vi "VanoceVanoce.vi"(11 "NXT/EV3":T1) -> (3 "NXT/EV3 2":T1)   [LabVIEW 2016]
uses:
  <vilib>/NXT/Subs/LVHSConnector.ctl
  <vilib>/NXT/LegoClasses/BrickReference/BrickReference.lvclass
  <vilib>/NXT/Block Support/NXT_OutputPort.ctl
  <vilib>/NXT/Dual Mode Library/Display/drawText_Center.vi
  <vilib>/NXT/Dual Mode Library/Sound/PlayC.vi
  <vilib>/NXT/Dual Mode Library/Sound/PlayA.vi
  <vilib>/NXT/Dual Mode Library/Sound/PlayG.vi
  <vilib>/NXT/Dual Mode Library/Sound/PlayE.vi
  <vilib>/NXT/Dual Mode Library/Sound/PlayD.vi
  <vilib>/NXT/Dual Mode Library/Waits/Wait_Num.vi
  <vilib>/NXT/Dual Mode Library/Sound/PlayB.vi
  <vilib>/NXT/Dual Mode Library/Sound/PlayF.vi
  <vilib>/NXT/Dual Mode Library/Sound/PlayFsharp.vi
  <vilib>/NXT/NXTIO Xnodes/NXTIONodeSubVIs/NXTMoveMotors.vi
  <vilib>/NXT/NXTIO Xnodes/NXTIONodeSubVIs/NXTStopMotors.vi
  <vilib>/NXT/NXTIO Xnodes/AddressXNode/NXTIOAddress.xnode
  <vilib>/NXT/NXTIO Xnodes/NXTIOXNode/NXTIO.xnode
panel:
  in  "Poèet opakování":i32
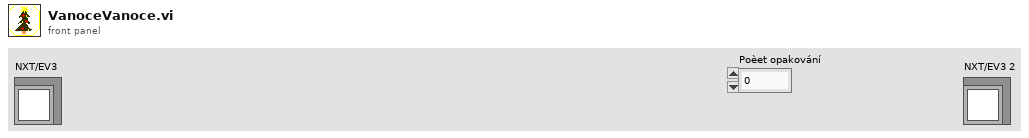
[diagram p1: front panel]
types:
  T1 = typedef "LVHSConnector.ctl" = refnum<class "BrickReference.lvclass">
  T2 = typedef "NXT_OutputPort.ctl" = u8
diagram:
  w8 = u16 5 items=["3"=3, "4"=4, "5"=5, "6"=6, "7"=7] ("Octave")
  w9 = u16 4 items=["3"=3, "4"=4, "5"=5, "6"=6, "7"=7] ("Octave")
  w10 = u16 4 items=["3"=3, "4"=4, "5"=5, "6"=6, "7"=7] ("Octave")
  w11 = u16 4 items=["3"=3, "4"=4, "5"=5, "6"=6, "7"=7] ("Octave")
  w21 = u16 4 items=["3"=3, "4"=4, "5"=5, "6"=6, "7"=7] ("Octave")
  w20 = u16 4 items=["3"=3, "4"=4, "5"=5, "6"=6, "7"=7] ("Octave")
  w48 = u16 4 items=["3"=3, "4"=4, "5"=5, "6"=6, "7"=7] ("Octave")
  w46 = u16 4 items=["3"=3, "4"=4, "5"=5, "6"=6, "7"=7] ("Octave")
  w41 = u16 4 items=["3"=3, "4"=4, "5"=5, "6"=6, "7"=7] ("Octave")
  w40 = u16 4 items=["3"=3, "4"=4, "5"=5, "6"=6, "7"=7] ("Octave")
  w35 = u16 4 items=["3"=3, "4"=4, "5"=5, "6"=6, "7"=7] ("Octave")
  w34 = u16 4 items=["3"=3, "4"=4, "5"=5, "6"=6, "7"=7] ("Octave")
  w33 = u16 4 items=["3"=3, "4"=4, "5"=5, "6"=6, "7"=7] ("Octave")
  w28 = u16 4 items=["3"=3, "4"=4, "5"=5, "6"=6, "7"=7] ("Octave")
  w25 = u16 5 items=["3"=3, "4"=4, "5"=5, "6"=6, "7"=7] ("Octave")
  w24 = u16 5 items=["3"=3, "4"=4, "5"=5, "6"=6, "7"=7] ("Octave")
  w53 = u16 4 items=["3"=3, "4"=4, "5"=5, "6"=6, "7"=7] ("Octave")
  w54 = u16 4 items=["3"=3, "4"=4, "5"=5, "6"=6, "7"=7] ("Octave")
  w55 = u16 4 items=["3"=3, "4"=4, "5"=5, "6"=6, "7"=7] ("Octave")
  w69 = u16 4 items=["3"=3, "4"=4, "5"=5, "6"=6, "7"=7] ("Octave")
  w70 = u16 4 items=["3"=3, "4"=4, "5"=5, "6"=6, "7"=7] ("Octave")
  w71 = u16 4 items=["3"=3, "4"=4, "5"=5, "6"=6, "7"=7] ("Octave")
  w72 = u16 4 items=["3"=3, "4"=4, "5"=5, "6"=6, "7"=7] ("Octave")
  w73 = u16 4 items=["3"=3, "4"=4, "5"=5, "6"=6, "7"=7] ("Octave")
  w74 = u16 4 items=["3"=3, "4"=4, "5"=5, "6"=6, "7"=7] ("Octave")
  w86 = u16 4 items=["3"=3, "4"=4, "5"=5, "6"=6, "7"=7] ("Octave")
  w88 = u16 4 items=["3"=3, "4"=4, "5"=5, "6"=6, "7"=7] ("Octave")
  w93 = u16 4 items=["3"=3, "4"=4, "5"=5, "6"=6, "7"=7] ("Octave")
  w94 = u16 4 items=["3"=3, "4"=4, "5"=5, "6"=6, "7"=7] ("Octave")
  w99 = u16 4 items=["3"=3, "4"=4, "5"=5, "6"=6, "7"=7] ("Octave")
  w100 = u16 4 items=["3"=3, "4"=4, "5"=5, "6"=6, "7"=7] ("Octave")
  w101 = u16 4 items=["3"=3, "4"=4, "5"=5, "6"=6, "7"=7] ("Octave")
  w107 = u16 4 items=["3"=3, "4"=4, "5"=5, "6"=6, "7"=7] ("Octave")
  w110 = u16 5 items=["3"=3, "4"=4, "5"=5, "6"=6, "7"=7] ("Octave")
  w111 = u16 5 items=["3"=3, "4"=4, "5"=5, "6"=6, "7"=7] ("Octave")
  w116 = u16 4 items=["3"=3, "4"=4, "5"=5, "6"=6, "7"=7] ("Octave")
  w119 = u16 4 items=["3"=3, "4"=4, "5"=5, "6"=6, "7"=7] ("Octave")
  w120 = u16 4 items=["3"=3, "4"=4, "5"=5, "6"=6, "7"=7] ("Octave")
  w146 = u16 4 items=["3"=3, "4"=4, "5"=5, "6"=6, "7"=7] ("Octave")
  w150 = u16 4 items=["3"=3, "4"=4, "5"=5, "6"=6, "7"=7] ("Octave")
  w147 = u16 4 items=["3"=3, "4"=4, "5"=5, "6"=6, "7"=7] ("Octave")
  w139 = u16 4 items=["3"=3, "4"=4, "5"=5, "6"=6, "7"=7] ("Octave")
  w136 = u16 4 items=["3"=3, "4"=4, "5"=5, "6"=6, "7"=7] ("Octave")
  w131 = u16 4 items=["3"=3, "4"=4, "5"=5, "6"=6, "7"=7] ("Octave")
  w134 = u16 4 items=["3"=3, "4"=4, "5"=5, "6"=6, "7"=7] ("Octave")
  w126 = u16 4 items=["3"=3, "4"=4, "5"=5, "6"=6, "7"=7] ("Octave")
  w123 = u16 4 items=["3"=3, "4"=4, "5"=5, "6"=6, "7"=7] ("Octave")
  w122 = u16 4 items=["3"=3, "4"=4, "5"=5, "6"=6, "7"=7] ("Octave")
  w168 = u16 4 items=["3"=3, "4"=4, "5"=5, "6"=6, "7"=7] ("Octave")
  w165 = u16 4 items=["3"=3, "4"=4, "5"=5, "6"=6, "7"=7] ("Octave")
  w161 = u16 4 items=["3"=3, "4"=4, "5"=5, "6"=6, "7"=7] ("Octave")
  w164 = u16 4 items=["3"=3, "4"=4, "5"=5, "6"=6, "7"=7] ("Octave")
  w176 = u16 4 items=["3"=3, "4"=4, "5"=5, "6"=6, "7"=7] ("Octave")
  w179 = u16 4 items=["3"=3, "4"=4, "5"=5, "6"=6, "7"=7] ("Octave")
  w184 = u16 4 items=["3"=3, "4"=4, "5"=5, "6"=6, "7"=7] ("Octave")
  w181 = u16 4 items=["3"=3, "4"=4, "5"=5, "6"=6, "7"=7] ("Octave")
  w189 = u16 4 items=["3"=3, "4"=4, "5"=5, "6"=6, "7"=7] ("Octave")
  w192 = u16 4 items=["3"=3, "4"=4, "5"=5, "6"=6, "7"=7] ("Octave")
  w193 = u16 4 items=["3"=3, "4"=4, "5"=5, "6"=6, "7"=7] ("Octave")
  w196 = u16 4 items=["3"=3, "4"=4, "5"=5, "6"=6, "7"=7] ("Octave")
  w204 = u16 5 items=["3"=3, "4"=4, "5"=5, "6"=6, "7"=7] ("Octave")
  w205 = u16 4 items=["3"=3, "4"=4, "5"=5, "6"=6, "7"=7] ("Octave")
  w206 = u16 4 items=["3"=3, "4"=4, "5"=5, "6"=6, "7"=7] ("Octave")
  w207 = u16 4 items=["3"=3, "4"=4, "5"=5, "6"=6, "7"=7] ("Octave")
  w217 = u16 4 items=["3"=3, "4"=4, "5"=5, "6"=6, "7"=7] ("Octave")
  w216 = u16 4 items=["3"=3, "4"=4, "5"=5, "6"=6, "7"=7] ("Octave")
  w244 = u16 4 items=["3"=3, "4"=4, "5"=5, "6"=6, "7"=7] ("Octave")
  w242 = u16 4 items=["3"=3, "4"=4, "5"=5, "6"=6, "7"=7] ("Octave")
  w237 = u16 4 items=["3"=3, "4"=4, "5"=5, "6"=6, "7"=7] ("Octave")
  w236 = u16 4 items=["3"=3, "4"=4, "5"=5, "6"=6, "7"=7] ("Octave")
  w231 = u16 4 items=["3"=3, "4"=4, "5"=5, "6"=6, "7"=7] ("Octave")
  w230 = u16 4 items=["3"=3, "4"=4, "5"=5, "6"=6, "7"=7] ("Octave")
  w229 = u16 4 items=["3"=3, "4"=4, "5"=5, "6"=6, "7"=7] ("Octave")
  w224 = u16 4 items=["3"=3, "4"=4, "5"=5, "6"=6, "7"=7] ("Octave")
  w221 = u16 5 items=["3"=3, "4"=4, "5"=5, "6"=6, "7"=7] ("Octave")
  w220 = u16 5 items=["3"=3, "4"=4, "5"=5, "6"=6, "7"=7] ("Octave")
  w249 = u16 4 items=["3"=3, "4"=4, "5"=5, "6"=6, "7"=7] ("Octave")
  w250 = u16 4 items=["3"=3, "4"=4, "5"=5, "6"=6, "7"=7] ("Octave")
  w251 = u16 4 items=["3"=3, "4"=4, "5"=5, "6"=6, "7"=7] ("Octave")
  w265 = u16 4 items=["3"=3, "4"=4, "5"=5, "6"=6, "7"=7] ("Octave")
  w266 = u16 4 items=["3"=3, "4"=4, "5"=5, "6"=6, "7"=7] ("Octave")
  w267 = u16 4 items=["3"=3, "4"=4, "5"=5, "6"=6, "7"=7] ("Octave")
  w268 = u16 4 items=["3"=3, "4"=4, "5"=5, "6"=6, "7"=7] ("Octave")
  w269 = u16 4 items=["3"=3, "4"=4, "5"=5, "6"=6, "7"=7] ("Octave")
  w270 = u16 4 items=["3"=3, "4"=4, "5"=5, "6"=6, "7"=7] ("Octave")
  w280 = i16 5 items=["1", "2", "3", "4", "5", "6", "7", "8", "9", "10", "11", "12"] ("Line")
  w284 = u16 4 items=["3"=3, "4"=4, "5"=5, "6"=6, "7"=7] ("Octave")
  w286 = u16 4 items=["3"=3, "4"=4, "5"=5, "6"=6, "7"=7] ("Octave")
  w291 = u16 4 items=["3"=3, "4"=4, "5"=5, "6"=6, "7"=7] ("Octave")
  w292 = u16 4 items=["3"=3, "4"=4, "5"=5, "6"=6, "7"=7] ("Octave")
  w297 = u16 4 items=["3"=3, "4"=4, "5"=5, "6"=6, "7"=7] ("Octave")
  w298 = u16 4 items=["3"=3, "4"=4, "5"=5, "6"=6, "7"=7] ("Octave")
  w299 = u16 4 items=["3"=3, "4"=4, "5"=5, "6"=6, "7"=7] ("Octave")
  w305 = u16 4 items=["3"=3, "4"=4, "5"=5, "6"=6, "7"=7] ("Octave")
  w308 = u16 5 items=["3"=3, "4"=4, "5"=5, "6"=6, "7"=7] ("Octave")
  w309 = u16 5 items=["3"=3, "4"=4, "5"=5, "6"=6, "7"=7] ("Octave")
  n1 = for {
    N: "Poèet opakování" -> [_]
    n2 = xnode "Motors"() -> ("Motor"=w313:cluster{"Port":T2, "Port":T2})
    n3 = xnode "Move Motors"("Power/Speed 2"=i8 -75, "Power/Speed 1"=i8 75, "Motors"=w313) -> ("NXT/EV3"=w328:T1)  [unwired: 1 in]
    n4 = call-poly <vilib>:"PolyWait.vi"("Time (1 sec)"=sgl 0.5, "NXT/EV3"=w328) -> ("NXT/EV3"=w327:T1)  [unwired: 2 in]
    n5 = xnode "Stop Motors"("Motors"=w313, "NXT/EV3"=w327) -> ("NXT/EV3"=w319:T1)
    n6 = xnode "Move Motors"("Power/Speed 2"=i8 75, "Power/Speed 1"=i8 -75, "Motors"=w313, "NXT/EV3"=w319) -> ("NXT/EV3"=w320:T1)
    n7 = call-poly <vilib>:"PolyWait.vi"("Time (1 sec)"=sgl 0.5, "NXT/EV3"=w320) -> ("NXT/EV3"=w321:T1)  [unwired: 2 in]
    n8 = xnode "Stop Motors"("Motors"=w313, "NXT/EV3"=w321) -> ("NXT/EV3"=w312:T1)
    n9 = xnode "Move Motors"("Power/Speed 2"=i8 20, "Power/Speed 1"=i8 20, "Motors"=w313, "NXT/EV3"=w312) -> ("NXT/EV3"=w317:T1)
    n10 = call-poly <vilib>:"PolyWait.vi"("Time (1 sec)"=sgl 0.5, "NXT/EV3"=w317) -> ("NXT/EV3"=w316:T1)  [unwired: 2 in]
    n11 = xnode "Stop Motors"("Motors"=w313, "NXT/EV3"=w316) -> ()  [unwired: 1 out]
  }
  n12 = call-poly <vilib>:"PolyDisplay.vi"("Text"="EV3 JUK3BOX:\nVanoce, Vanoce\n", "NXT/EV3"="NXT/EV3", "Line"=w280) -> ("NXT/EV3"=w197:T1)  [unwired: 1 in]
  n13 = call-poly <vilib>:"PolySound.vi"("Duration (500 ms)"=u16 1000, "NXT/EV3"=w197, "Octave"=w309) -> ("NXT/EV3"=w304:T1)  [unwired: 1 in]
  n14 = call-poly <vilib>:"PolySound.vi"("Duration (500 ms)"=u16 500, "NXT/EV3"=w304, "Octave"=w308) -> ("NXT/EV3"=w303:T1)  [unwired: 1 in]
  n15 = call-poly <vilib>:"PolySound.vi"("Duration (500 ms)"=u16 500, "NXT/EV3"=w303, "Octave"=w305) -> ("NXT/EV3"=w302:T1)  [unwired: 1 in]
  n16 = call-poly <vilib>:"PolySound.vi"("Duration (500 ms)"=u16 1000, "NXT/EV3"=w302, "Octave"=w299) -> ("NXT/EV3"=w301:T1)  [unwired: 1 in]
  n17 = call-poly <vilib>:"PolySound.vi"("Duration (500 ms)"=u16 500, "NXT/EV3"=w301, "Octave"=w298) -> ("NXT/EV3"=w300:T1)  [unwired: 1 in]
  n18 = call-poly <vilib>:"PolySound.vi"("Duration (500 ms)"=u16 500, "NXT/EV3"=w300, "Octave"=w297) -> ("NXT/EV3"=w289:T1)  [unwired: 1 in]
  n19 = call-poly <vilib>:"PolySound.vi"("Duration (500 ms)"=u16 500, "NXT/EV3"=w289, "Octave"=w292) -> ("NXT/EV3"=w288:T1)  [unwired: 1 in]
  n20 = call-poly <vilib>:"PolySound.vi"("Duration (500 ms)"=u16 1000, "NXT/EV3"=w288, "Octave"=w291) -> ("NXT/EV3"=w285:T1)  [unwired: 1 in]
  n21 = call-poly <vilib>:"PolySound.vi"("Duration (500 ms)"=u16 500, "NXT/EV3"=w285, "Octave"=w286) -> ("NXT/EV3"=w283:T1)  [unwired: 1 in]
  n22 = call-poly <vilib>:"PolySound.vi"("Duration (500 ms)"=u16 1000, "NXT/EV3"=w283, "Octave"=w284) -> ("NXT/EV3"=w262:T1)  [unwired: 1 in]
  n23 = call-poly <vilib>:"PolyWait.vi"("Time (1 sec)"=sgl 0.7, "NXT/EV3"=w262) -> ("NXT/EV3"=w261:T1)  [unwired: 2 in]
  n24 = call-poly <vilib>:"PolySound.vi"("Duration (500 ms)"=u16 500, "NXT/EV3"=w261, "Octave"=w270) -> ("NXT/EV3"=w279:T1)  [unwired: 1 in]
  n25 = call-poly <vilib>:"PolySound.vi"("Duration (500 ms)"=u16 1000, "NXT/EV3"=w279, "Octave"=w269) -> ("NXT/EV3"=w278:T1)  [unwired: 1 in]
  n26 = call-poly <vilib>:"PolySound.vi"("Duration (500 ms)"=u16 500, "NXT/EV3"=w278, "Octave"=w268) -> ("NXT/EV3"=w277:T1)  [unwired: 1 in]
  n27 = call-poly <vilib>:"PolySound.vi"("Duration (500 ms)"=u16 1000, "NXT/EV3"=w277, "Octave"=w267) -> ("NXT/EV3"=w276:T1)  [unwired: 1 in]
  n28 = call-poly <vilib>:"PolySound.vi"("Duration (500 ms)"=u16 1000, "NXT/EV3"=w276, "Octave"=w266) -> ("NXT/EV3"=w263:T1)  [unwired: 1 in]
  n29 = call-poly <vilib>:"PolySound.vi"("Duration (500 ms)"=u16 1900, "NXT/EV3"=w263, "Octave"=w265) -> ("NXT/EV3"=w259:T1)  [unwired: 1 in]
  n30 = call-poly <vilib>:"PolyWait.vi"("Time (1 sec)"=sgl 0.3, "NXT/EV3"=w259) -> ("NXT/EV3"=w257:T1)  [unwired: 2 in]
  n31 = call-poly <vilib>:"PolySound.vi"("Duration (500 ms)"=u16 500, "NXT/EV3"=w257, "Octave"=w251) -> ("NXT/EV3"=w256:T1)  [unwired: 1 in]
  n32 = call-poly <vilib>:"PolySound.vi"("Duration (500 ms)"=u16 500, "NXT/EV3"=w256, "Octave"=w250) -> ("NXT/EV3"=w255:T1)  [unwired: 1 in]
  n33 = call-poly <vilib>:"PolySound.vi"("Duration (500 ms)"=u16 500, "NXT/EV3"=w255, "Octave"=w249) -> ("NXT/EV3"=w218:T1)  [unwired: 1 in]
  n34 = call-poly <vilib>:"PolySound.vi"("Duration (500 ms)"=u16 1000, "NXT/EV3"=w218, "Octave"=w220) -> ("NXT/EV3"=w225:T1)  [unwired: 1 in]
  n35 = call-poly <vilib>:"PolySound.vi"("Duration (500 ms)"=u16 500, "NXT/EV3"=w225, "Octave"=w221) -> ("NXT/EV3"=w198:T1)  [unwired: 1 in]
  "NXT/EV3 2" <- w198
  n36 = call-poly <vilib>:"PolySound.vi"("Duration (500 ms)"=u16 500, "NXT/EV3"=w198, "Octave"=w224) -> ("NXT/EV3"=w226:T1)  [unwired: 1 in]
  n37 = call-poly <vilib>:"PolySound.vi"("Duration (500 ms)"=u16 1000, "NXT/EV3"=w226, "Octave"=w229) -> ("NXT/EV3"=w227:T1)  [unwired: 1 in]
  n38 = call-poly <vilib>:"PolySound.vi"("Duration (500 ms)"=u16 500, "NXT/EV3"=w227, "Octave"=w230) -> ("NXT/EV3"=w228:T1)  [unwired: 1 in]
  n39 = call-poly <vilib>:"PolySound.vi"("Duration (500 ms)"=u16 500, "NXT/EV3"=w228, "Octave"=w231) -> ("NXT/EV3"=w239:T1)  [unwired: 1 in]
  n40 = call-poly <vilib>:"PolySound.vi"("Duration (500 ms)"=u16 500, "NXT/EV3"=w239, "Octave"=w236) -> ("NXT/EV3"=w240:T1)  [unwired: 1 in]
  n41 = call-poly <vilib>:"PolySound.vi"("Duration (500 ms)"=u16 1000, "NXT/EV3"=w240, "Octave"=w237) -> ("NXT/EV3"=w243:T1)  [unwired: 1 in]
  n42 = call-poly <vilib>:"PolySound.vi"("Duration (500 ms)"=u16 500, "NXT/EV3"=w243, "Octave"=w242) -> ("NXT/EV3"=w245:T1)  [unwired: 1 in]
  n43 = call-poly <vilib>:"PolySound.vi"("Duration (500 ms)"=u16 1000, "NXT/EV3"=w245, "Octave"=w244) -> ("NXT/EV3"=w247:T1)  [unwired: 1 in]
  n44 = call-poly <vilib>:"PolyWait.vi"("Time (1 sec)"=sgl 0.7, "NXT/EV3"=w247) -> ("NXT/EV3"=w212:T1)  [unwired: 2 in]
  n45 = call-poly <vilib>:"PolySound.vi"("Duration (500 ms)"=u16 500, "NXT/EV3"=w212, "Octave"=w216) -> ("NXT/EV3"=w213:T1)  [unwired: 1 in]
  n46 = call-poly <vilib>:"PolySound.vi"("Duration (500 ms)"=u16 1000, "NXT/EV3"=w213, "Octave"=w217) -> ("NXT/EV3"=w211:T1)  [unwired: 1 in]
  n47 = call-poly <vilib>:"PolySound.vi"("Duration (500 ms)"=u16 500, "NXT/EV3"=w211, "Octave"=w207) -> ("NXT/EV3"=w210:T1)  [unwired: 1 in]
  n48 = call-poly <vilib>:"PolySound.vi"("Duration (500 ms)"=u16 1000, "NXT/EV3"=w210, "Octave"=w206) -> ("NXT/EV3"=w209:T1)  [unwired: 1 in]
  n49 = call-poly <vilib>:"PolySound.vi"("Duration (500 ms)"=u16 1000, "NXT/EV3"=w209, "Octave"=w205) -> ("NXT/EV3"=w208:T1)  [unwired: 1 in]
  n50 = call-poly <vilib>:"PolySound.vi"("Duration (500 ms)"=u16 2000, "NXT/EV3"=w208, "Octave"=w204) -> ("NXT/EV3"=w173:T1)  [unwired: 1 in]
  n51 = call-poly <vilib>:"PolyWait.vi"("Time (1 sec)"=sgl 0.7, "NXT/EV3"=w173) -> ("NXT/EV3"=w172:T1)  [unwired: 2 in]
  n52 = call-poly <vilib>:"PolySound.vi"("Duration (500 ms)"=u16 500, "NXT/EV3"=w172, "Octave"=w196) -> ("NXT/EV3"=w188:T1)  [unwired: 1 in]
  n53 = call-poly <vilib>:"PolySound.vi"("Duration (500 ms)"=u16 500, "NXT/EV3"=w188, "Octave"=w193) -> ("NXT/EV3"=w187:T1)  [unwired: 1 in]
  n54 = call-poly <vilib>:"PolySound.vi"("Duration (500 ms)"=u16 500, "NXT/EV3"=w187, "Octave"=w192) -> ("NXT/EV3"=w186:T1)  [unwired: 1 in]
  n55 = call-poly <vilib>:"PolySound.vi"("Duration (500 ms)"=u16 500, "NXT/EV3"=w186, "Octave"=w189) -> ("NXT/EV3"=w180:T1)  [unwired: 1 in]
  n56 = call-poly <vilib>:"PolySound.vi"("Duration (500 ms)"=u16 500, "NXT/EV3"=w180, "Octave"=w181) -> ("NXT/EV3"=w185:T1)  [unwired: 1 in]
  n57 = call-poly <vilib>:"PolySound.vi"("Duration (500 ms)"=u16 500, "NXT/EV3"=w185, "Octave"=w184) -> ("NXT/EV3"=w174:T1)  [unwired: 1 in]
  n58 = call-poly <vilib>:"PolySound.vi"("Duration (500 ms)"=u16 500, "NXT/EV3"=w174, "Octave"=w179) -> ("NXT/EV3"=w175:T1)  [unwired: 1 in]
  n59 = call-poly <vilib>:"PolySound.vi"("Duration (500 ms)"=u16 500, "NXT/EV3"=w175, "Octave"=w176) -> ("NXT/EV3"=w159:T1)  [unwired: 1 in]
  n60 = call-poly <vilib>:"PolySound.vi"("Duration (500 ms)"=u16 500, "NXT/EV3"=w159, "Octave"=w164) -> ("NXT/EV3"=w160:T1)  [unwired: 1 in]
  n61 = call-poly <vilib>:"PolySound.vi"("Duration (500 ms)"=u16 500, "NXT/EV3"=w160, "Octave"=w161) -> ("NXT/EV3"=w170:T1)  [unwired: 1 in]
  n62 = call-poly <vilib>:"PolySound.vi"("Duration (500 ms)"=u16 500, "NXT/EV3"=w170, "Octave"=w165) -> ("NXT/EV3"=w169:T1)  [unwired: 1 in]
  n63 = call-poly <vilib>:"PolySound.vi"("Duration (500 ms)"=u16 500, "NXT/EV3"=w169, "Octave"=w168) -> ("NXT/EV3"=w158:T1)  [unwired: 1 in]
  n64 = call-poly <vilib>:"PolySound.vi"("Duration (500 ms)"=u16 500, "NXT/EV3"=w158) -> ("NXT/EV3"=w157:T1)  [unwired: 2 in]
  n65 = call-poly <vilib>:"PolySound.vi"("Duration (500 ms)"=u16 500, "NXT/EV3"=w157) -> ("NXT/EV3"=w156:T1)  [unwired: 2 in]
  n66 = call-poly <vilib>:"PolySound.vi"("Duration (500 ms)"=u16 750, "NXT/EV3"=w156) -> ("NXT/EV3"=w118:T1)  [unwired: 2 in]
  n67 = call-poly <vilib>:"PolySound.vi"("NXT/EV3"=w118, "Octave"=w119) -> ("NXT/EV3"=w127:T1)  [unwired: 2 in]
  n68 = call-poly <vilib>:"PolySound.vi"("Duration (500 ms)"=u16 500, "NXT/EV3"=w127, "Octave"=w122) -> ("NXT/EV3"=w128:T1)  [unwired: 1 in]
  n69 = call-poly <vilib>:"PolySound.vi"("Duration (500 ms)"=u16 500, "NXT/EV3"=w128, "Octave"=w123) -> ("NXT/EV3"=w129:T1)  [unwired: 1 in]
  n70 = call-poly <vilib>:"PolySound.vi"("Duration (500 ms)"=u16 500, "NXT/EV3"=w129, "Octave"=w126) -> ("NXT/EV3"=w135:T1)  [unwired: 1 in]
  n71 = call-poly <vilib>:"PolySound.vi"("Duration (500 ms)"=u16 500, "NXT/EV3"=w135, "Octave"=w134) -> ("NXT/EV3"=w130:T1)  [unwired: 1 in]
  n72 = call-poly <vilib>:"PolySound.vi"("Duration (500 ms)"=u16 500, "NXT/EV3"=w130, "Octave"=w131) -> ("NXT/EV3"=w141:T1)  [unwired: 1 in]
  n73 = call-poly <vilib>:"PolySound.vi"("Duration (500 ms)"=u16 500, "NXT/EV3"=w141, "Octave"=w136) -> ("NXT/EV3"=w140:T1)  [unwired: 1 in]
  n74 = call-poly <vilib>:"PolySound.vi"("Duration (500 ms)"=u16 500, "NXT/EV3"=w140, "Octave"=w139) -> ("NXT/EV3"=w152:T1)  [unwired: 1 in]
  n75 = call-poly <vilib>:"PolySound.vi"("Duration (500 ms)"=u16 500, "NXT/EV3"=w152, "Octave"=w147) -> ("NXT/EV3"=w151:T1)  [unwired: 1 in]
  n76 = call-poly <vilib>:"PolySound.vi"("Duration (500 ms)"=u16 500, "NXT/EV3"=w151, "Octave"=w150) -> ("NXT/EV3"=w142:T1)  [unwired: 1 in]
  n77 = call-poly <vilib>:"PolySound.vi"("Duration (500 ms)"=u16 500, "NXT/EV3"=w142, "Octave"=w146) -> ("NXT/EV3"=w143:T1)  [unwired: 1 in]
  n78 = call-poly <vilib>:"PolySound.vi"("Duration (500 ms)"=u16 500, "NXT/EV3"=w143, "Octave"=w120) -> ("NXT/EV3"=w115:T1)  [unwired: 1 in]
  n79 = call-poly <vilib>:"PolySound.vi"("Duration (500 ms)"=u16 750, "NXT/EV3"=w115, "Octave"=w116) -> ("NXT/EV3"=w114:T1)  [unwired: 1 in]
  n80 = call-poly <vilib>:"PolyWait.vi"("Time (1 sec)"=sgl 0.75, "NXT/EV3"=w114) -> ("NXT/EV3"=w2:T1)  [unwired: 2 in]
  n81 = call-poly <vilib>:"PolySound.vi"("Duration (500 ms)"=u16 1000, "NXT/EV3"=w2, "Octave"=w111) -> ("NXT/EV3"=w106:T1)  [unwired: 1 in]
  n82 = call-poly <vilib>:"PolySound.vi"("Duration (500 ms)"=u16 500, "NXT/EV3"=w106, "Octave"=w110) -> ("NXT/EV3"=w105:T1)  [unwired: 1 in]
  n83 = call-poly <vilib>:"PolySound.vi"("Duration (500 ms)"=u16 500, "NXT/EV3"=w105, "Octave"=w107) -> ("NXT/EV3"=w104:T1)  [unwired: 1 in]
  n84 = call-poly <vilib>:"PolySound.vi"("Duration (500 ms)"=u16 1000, "NXT/EV3"=w104, "Octave"=w101) -> ("NXT/EV3"=w103:T1)  [unwired: 1 in]
  n85 = call-poly <vilib>:"PolySound.vi"("Duration (500 ms)"=u16 500, "NXT/EV3"=w103, "Octave"=w100) -> ("NXT/EV3"=w102:T1)  [unwired: 1 in]
  n86 = call-poly <vilib>:"PolySound.vi"("Duration (500 ms)"=u16 500, "NXT/EV3"=w102, "Octave"=w99) -> ("NXT/EV3"=w91:T1)  [unwired: 1 in]
  n87 = call-poly <vilib>:"PolySound.vi"("Duration (500 ms)"=u16 500, "NXT/EV3"=w91, "Octave"=w94) -> ("NXT/EV3"=w90:T1)  [unwired: 1 in]
  n88 = call-poly <vilib>:"PolySound.vi"("Duration (500 ms)"=u16 1000, "NXT/EV3"=w90, "Octave"=w93) -> ("NXT/EV3"=w87:T1)  [unwired: 1 in]
  n89 = call-poly <vilib>:"PolySound.vi"("Duration (500 ms)"=u16 500, "NXT/EV3"=w87, "Octave"=w88) -> ("NXT/EV3"=w85:T1)  [unwired: 1 in]
  n90 = call-poly <vilib>:"PolySound.vi"("Duration (500 ms)"=u16 1000, "NXT/EV3"=w85, "Octave"=w86) -> ("NXT/EV3"=w66:T1)  [unwired: 1 in]
  n91 = call-poly <vilib>:"PolyWait.vi"("Time (1 sec)"=sgl 0.7, "NXT/EV3"=w66) -> ("NXT/EV3"=w65:T1)  [unwired: 2 in]
  n92 = call-poly <vilib>:"PolySound.vi"("Duration (500 ms)"=u16 500, "NXT/EV3"=w65, "Octave"=w74) -> ("NXT/EV3"=w83:T1)  [unwired: 1 in]
  n93 = call-poly <vilib>:"PolySound.vi"("Duration (500 ms)"=u16 1000, "NXT/EV3"=w83, "Octave"=w73) -> ("NXT/EV3"=w82:T1)  [unwired: 1 in]
  n94 = call-poly <vilib>:"PolySound.vi"("Duration (500 ms)"=u16 500, "NXT/EV3"=w82, "Octave"=w72) -> ("NXT/EV3"=w81:T1)  [unwired: 1 in]
  n95 = call-poly <vilib>:"PolySound.vi"("Duration (500 ms)"=u16 1000, "NXT/EV3"=w81, "Octave"=w71) -> ("NXT/EV3"=w80:T1)  [unwired: 1 in]
  n96 = call-poly <vilib>:"PolySound.vi"("Duration (500 ms)"=u16 1000, "NXT/EV3"=w80, "Octave"=w70) -> ("NXT/EV3"=w67:T1)  [unwired: 1 in]
  n97 = call-poly <vilib>:"PolySound.vi"("Duration (500 ms)"=u16 1900, "NXT/EV3"=w67, "Octave"=w69) -> ("NXT/EV3"=w63:T1)  [unwired: 1 in]
  n98 = call-poly <vilib>:"PolyWait.vi"("Time (1 sec)"=sgl 0.3, "NXT/EV3"=w63) -> ("NXT/EV3"=w61:T1)  [unwired: 2 in]
  n99 = call-poly <vilib>:"PolySound.vi"("Duration (500 ms)"=u16 500, "NXT/EV3"=w61, "Octave"=w55) -> ("NXT/EV3"=w60:T1)  [unwired: 1 in]
  n100 = call-poly <vilib>:"PolySound.vi"("Duration (500 ms)"=u16 500, "NXT/EV3"=w60, "Octave"=w54) -> ("NXT/EV3"=w59:T1)  [unwired: 1 in]
  n101 = call-poly <vilib>:"PolySound.vi"("Duration (500 ms)"=u16 500, "NXT/EV3"=w59, "Octave"=w53) -> ("NXT/EV3"=w22:T1)  [unwired: 1 in]
  n102 = call-poly <vilib>:"PolySound.vi"("Duration (500 ms)"=u16 1000, "NXT/EV3"=w22, "Octave"=w24) -> ("NXT/EV3"=w29:T1)  [unwired: 1 in]
  n103 = call-poly <vilib>:"PolySound.vi"("Duration (500 ms)"=u16 500, "NXT/EV3"=w29, "Octave"=w25) -> ("NXT/EV3"=w3:T1)  [unwired: 1 in]
  n104 = call-poly <vilib>:"PolySound.vi"("Duration (500 ms)"=u16 500, "NXT/EV3"=w3, "Octave"=w28) -> ("NXT/EV3"=w30:T1)  [unwired: 1 in]
  n105 = call-poly <vilib>:"PolySound.vi"("Duration (500 ms)"=u16 1000, "NXT/EV3"=w30, "Octave"=w33) -> ("NXT/EV3"=w31:T1)  [unwired: 1 in]
  n106 = call-poly <vilib>:"PolySound.vi"("Duration (500 ms)"=u16 500, "NXT/EV3"=w31, "Octave"=w34) -> ("NXT/EV3"=w32:T1)  [unwired: 1 in]
  n107 = call-poly <vilib>:"PolySound.vi"("Duration (500 ms)"=u16 500, "NXT/EV3"=w32, "Octave"=w35) -> ("NXT/EV3"=w43:T1)  [unwired: 1 in]
  n108 = call-poly <vilib>:"PolySound.vi"("Duration (500 ms)"=u16 500, "NXT/EV3"=w43, "Octave"=w40) -> ("NXT/EV3"=w44:T1)  [unwired: 1 in]
  n109 = call-poly <vilib>:"PolySound.vi"("Duration (500 ms)"=u16 1000, "NXT/EV3"=w44, "Octave"=w41) -> ("NXT/EV3"=w47:T1)  [unwired: 1 in]
  n110 = call-poly <vilib>:"PolySound.vi"("Duration (500 ms)"=u16 500, "NXT/EV3"=w47, "Octave"=w46) -> ("NXT/EV3"=w49:T1)  [unwired: 1 in]
  n111 = call-poly <vilib>:"PolySound.vi"("Duration (500 ms)"=u16 1000, "NXT/EV3"=w49, "Octave"=w48) -> ("NXT/EV3"=w51:T1)  [unwired: 1 in]
  n112 = call-poly <vilib>:"PolyWait.vi"("Time (1 sec)"=sgl 0.7, "NXT/EV3"=w51) -> ("NXT/EV3"=w16:T1)  [unwired: 2 in]
  n113 = call-poly <vilib>:"PolySound.vi"("Duration (500 ms)"=u16 500, "NXT/EV3"=w16, "Octave"=w20) -> ("NXT/EV3"=w17:T1)  [unwired: 1 in]
  n114 = call-poly <vilib>:"PolySound.vi"("Duration (500 ms)"=u16 1000, "NXT/EV3"=w17, "Octave"=w21) -> ("NXT/EV3"=w15:T1)  [unwired: 1 in]
  n115 = call-poly <vilib>:"PolySound.vi"("Duration (500 ms)"=u16 500, "NXT/EV3"=w15, "Octave"=w11) -> ("NXT/EV3"=w14:T1)  [unwired: 1 in]
  n116 = call-poly <vilib>:"PolySound.vi"("Duration (500 ms)"=u16 1000, "NXT/EV3"=w14, "Octave"=w10) -> ("NXT/EV3"=w13:T1)  [unwired: 1 in]
  n117 = call-poly <vilib>:"PolySound.vi"("Duration (500 ms)"=u16 1000, "NXT/EV3"=w13, "Octave"=w9) -> ("NXT/EV3"=w12:T1)  [unwired: 1 in]
  n118 = call-poly <vilib>:"PolySound.vi"("Duration (500 ms)"=u16 2000, "NXT/EV3"=w12, "Octave"=w8) -> ()  [unwired: 1 in, 1 out]
